vi "EnqueueManager (Array)__slk_QSM-PC (String).vi"(8 "error in (no error)":errorcluster, 9 "action (back)":enum16{"Back", "Front", "Replace"}(ring), 10 "elements":cluster{"State":string, "Data":variant}[](array[cluster]), 11 "queue in":refnum<queue>) -> (0 "error out":errorcluster)   [LabVIEW 2016, in "QSM-PC (String).lvlib"]
doc: "Sets elements to the different position of queue.\n\n<b>Functions:</b>\nEnqueue to the back of queue\nEnqueue to the front of queue\nReplace the elements of queue"
uses:
  Library/QSM-PC (String).lvlib
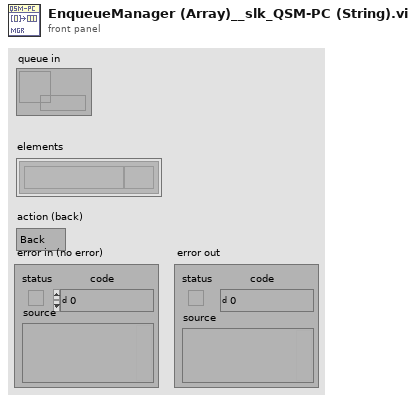
[diagram p1: front panel]
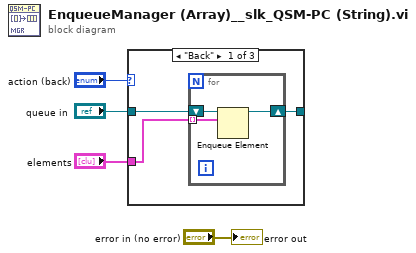
[diagram p0: block diagram]
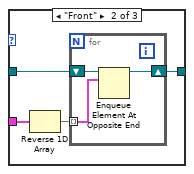
[diagram p2: hidden frame]
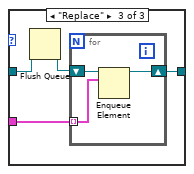
[diagram p3: hidden frame]
diagram:
  n1 = case shown="\"Back\"" "action (back)" {
    tunnel: "queue in" -> [w7 w14 w19]
    tunnel: "elements" -> [w6 w13 w20]
    tunnel: [w5 w12 w21] -> _
    frame "Back" {
      n2 = for {
        tunnel: w6 -> [w9] mode=indexing
        shift-right: [w8] -> w5
        shift-left: w7 -> [w10]
        n3 = Enqueue Element(queue=w10, element=w9) -> (queue out=w8:refnum<queue>)  [unwired: 1 in, 3 out]
      }
    }
    frame "Front" {
      n4 = Reverse 1D Array(array=w13) -> (reversed array=w11:cluster{"State":string, "Data":variant}[])
      n5 = for {
        tunnel: w11 -> [w16] mode=indexing
        shift-right: [w15] -> w12
        shift-left: w14 -> [w17]
        n6 = Enqueue Element At Opposite End(queue=w17, element=w16) -> (queue out=w15:refnum<queue>)  [unwired: 1 in, 3 out]
      }
    }
    frame "Replace" {
      n7 = Flush Queue(queue=w19) -> (queue out=w18:refnum<queue>)  [unwired: 1 in, 2 out]
      n8 = for {
        tunnel: w20 -> [w23] mode=indexing
        shift-right: [w22] -> w21
        shift-left: w18 -> [w24]
        n9 = Enqueue Element(queue=w24, element=w23) -> (queue out=w22:refnum<queue>)  [unwired: 1 in, 3 out]
      }
    }
  }
  "error out" <- "error in (no error)"
